vi "Calculator-teardown.vi"(8 "error in (no error)":errorcluster, 10 "result in":dbl, 11 "test case ID":string) -> (3 "result":bool)   [LabVIEW 2015]
doc: "The teardown VI should be executed after the VI under test in the harness VI. In this VI you can evaluate the outputs of the VI under test.\n\nSee the Help Document for more information. (<b>Help</b> > <b>IncQuery Labs</b> > <b>InstaCoverage</b> > <b>InstaCoverage Help...</b>)"
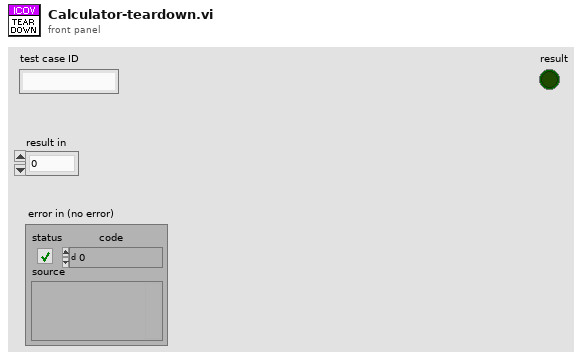
[diagram p1: front panel]
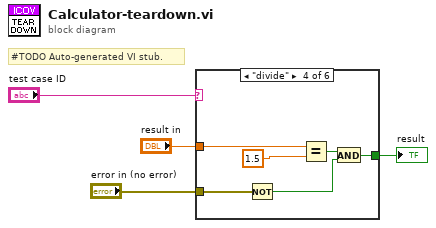
[diagram p0: block diagram]
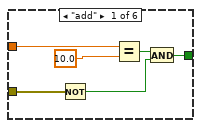
[diagram p2: hidden frame]
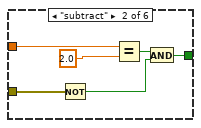
[diagram p3: hidden frame]
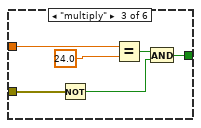
[diagram p4: hidden frame]
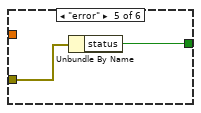
[diagram p5: hidden frame]
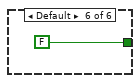
[diagram p6: hidden frame]
diagram:
  # "#TODO Auto-generated VI stub."
  n1 = case shown="\"divide\"" "test case ID" {
    tunnel: [w5 w11 w17 w23 w29 FALSE] -> w3
    tunnel: "result in" -> [w10 w16 w22 w28 _ _]
    tunnel: "error in (no error)" -> [w8 w14 w20 w26 w30 _]
    frame "add" {
      n2 = Not(x=w8) -> (.not. x?=w6:bool)
      n3 = Equal?(x=w10, y=10.0) -> (x = y?=w7:bool)
      n4 = And(x=w7, y=w6) -> (x .and. y?=w5:bool)
    }
    frame "subtract" {
      n5 = Not(x=w14) -> (.not. x?=w12:bool)
      n6 = Equal?(x=w16, y=2.0) -> (x = y?=w13:bool)
      n7 = And(x=w13, y=w12) -> (x .and. y?=w11:bool)
    }
    frame "multiply" {
      n8 = Not(x=w20) -> (.not. x?=w18:bool)
      n9 = Equal?(x=w22, y=24.0) -> (x = y?=w19:bool)
      n10 = And(x=w19, y=w18) -> (x .and. y?=w17:bool)
    }
    frame "divide" {
      n11 = Not(x=w26) -> (.not. x?=w24:bool)
      n12 = Equal?(x=w28, y=1.5) -> (x = y?=w25:bool)
      n13 = And(x=w25, y=w24) -> (x .and. y?=w23:bool)
    }
    frame "error" {
      n14 = Unbundle By Name(w30) -> ("status"=w29:bool)
    }
    frame Default {
    }
  }
  "result" <- w3
